vi "nodemcu_temp 00.vi"() -> ()   [LabVIEW 2018]
panel:
  out "웨이브폼 차트":dynamicdata(graph)
  out "Temp 2 (℃)":string
  out "온도2":dbl(graph)
  in  "문자열":string="http://192.168.137.202"
  out "Run":i32
  out "위치":path
  out "Data":string
  in  "불리언 2":bool=TRUE
  in  "Error In":errorcluster caption="에러 입력"
  out "Error Out":errorcluster caption="에러 출력"
  in  "정지 2":bool
  in  "Delay(s)":u32=4
  in  "188":bool=TRUE
  out "Temp 1 (℃)":string
  out "온도1":dbl(graph)
  in  "Clear":bool
  in  "정지":bool
  # "Temperture monitor"
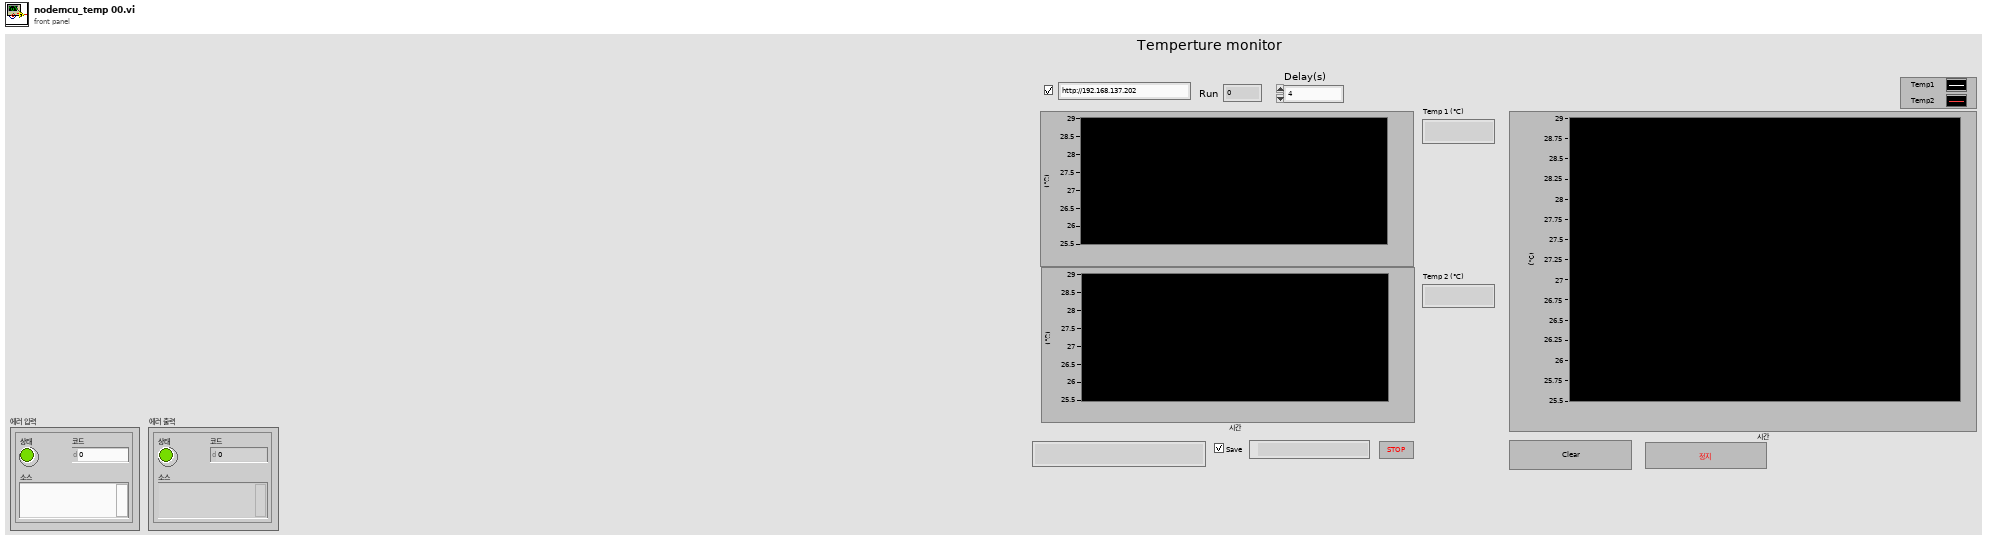
[diagram p1: front panel]
types:
  T1 = enum16{"Read", "Write", "ReadWrite", "BufferedRead", "BufferedReadWrite"}
  T2 = enum16{"open", "replace", "create", "open or create", "replace or create", "replace or create with confirmation"}
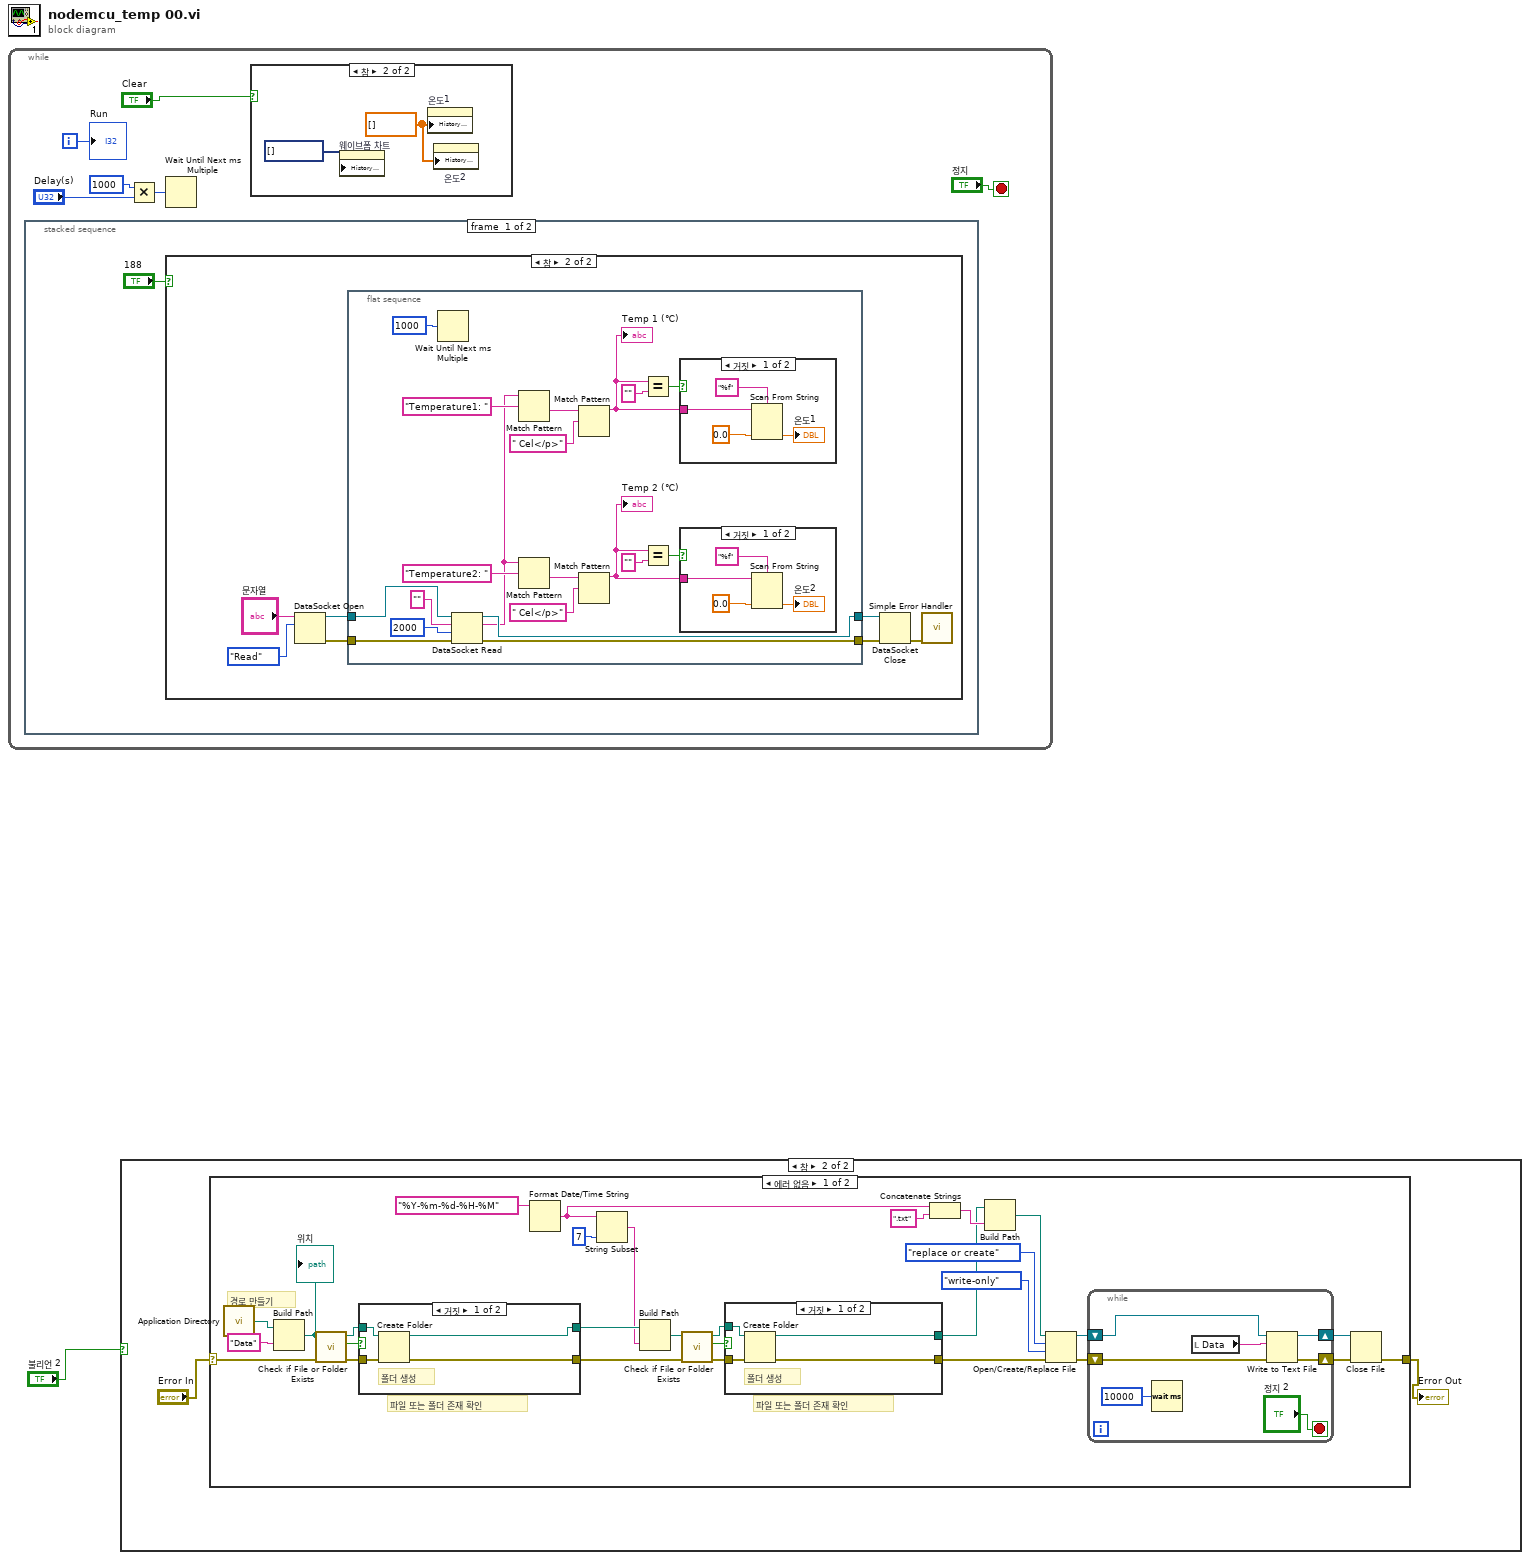
[diagram p0: block diagram]
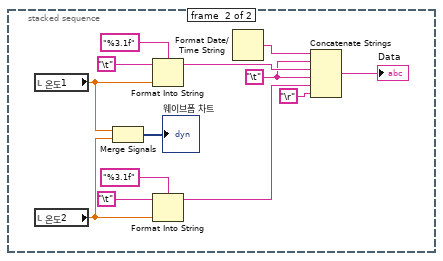
[diagram p10: hidden frame]
diagram:
  n1 = while {
    i -> [w5]
    stop <- "정지" stop-if-true
    n2 = stacked-sequence {
      frame #0 {
        n3 = case shown="참" "188" {
          frame False {
          }
          frame True {
            n4 = DataSocket Open(10:T1."Read" ("mode"), 11:"문자열") -> (0:w13:errorcluster, 3:w15:refnum<k13>)  [unwired: 2 in]
            n5 = flat-sequence {
              tunnel: w15 -> [w37]
              tunnel: [w36] -> w14
              tunnel: w13 -> [w35]
              tunnel: [w34] -> w12
              frame #0 {
                n6 = Wait Until Next ms Multiple(millisecond multiple=u32 1000 ("ms 배수")) -> ()  [unwired: 1 out]
                n7 = DataSocket Read(8:w35, 9:2000 ("ms 타임아웃(10000)"), 10:"", 11:w37) -> (0:w34:errorcluster, 2:w18:string, 3:w36:refnum<k13>)  [unwired: 1 in, 4 out]
                n8 = Match Pattern(string=w18, regular expression="Temperature1: " ("검색 문자열/문자 (-)")) -> (after substring=w33:string)  [unwired: 1 in, 3 out]
                n9 = Match Pattern(string=w18, regular expression="Temperature2: " ("검색 문자열/문자 (-)")) -> (after substring=w19:string)  [unwired: 1 in, 3 out]
                n10 = Match Pattern(string=w33, regular expression=" Cel</p>" ("정규식")) -> (before substring=w26:string)  [unwired: 1 in, 3 out]
                "Temp 1 (℃)" <- w26
                n11 = Match Pattern(string=w19, regular expression=" Cel</p>" ("정규식")) -> (before substring=w24:string)  [unwired: 1 in, 3 out]
                "Temp 2 (℃)" <- w24
                n12 = Equal?(x=w26, y="") -> (x = y?=w27:bool)
                n13 = Equal?(x=w24, y="") -> (x = y?=w23:bool)
                n14 = case shown="거짓" w27 {
                  tunnel: w26 -> [w42 _]
                  frame False {
                    n15 = Scan From String(format string="%f" ("포맷 문자열"), input string=w42, default 1=0.0 ("기본값 1")) -> (output 1=→"온도1":dbl)  [unwired: 2 in, 3 out]
                  }
                  frame True {
                  }
                }
                n16 = case shown="거짓" w23 {
                  tunnel: w24 -> [w38 _]
                  frame False {
                    n17 = Scan From String(format string="%f" ("포맷 문자열"), input string=w38, default 1=0.0 ("기본값 1")) -> (output 1=→"온도2":dbl)  [unwired: 2 in, 3 out]
                  }
                  frame True {
                  }
                }
              }
            }
            n18 = DataSocket Close(8:w12, 11:w14) -> (0:w16:errorcluster)  [unwired: 1 in, 1 out]
            n19 = call <vilib>:"Simple Error Handler.vi"("error in (no error)"=w16) -> ()  [unwired: 4 in, 5 out]
          }
        }
      }
      frame #1 {
        w49 = "\t"
        n20 = local read "온도1"() -> (w48:dbl)
        n21 = local read "온도2"() -> (w47:dbl)
        n22 = Merge Signals(w48, w47) -> (→"웨이브폼 차트":dynamicdata)
        n23 = Format Into String(format string="%3.1f" ("포맷 문자열"), initial string="\t", w48) -> (resulting string=w57:string)  [unwired: 1 in, 1 out]
        n24 = Format Into String(format string="%3.1f" ("포맷 문자열"), initial string="\t", w47) -> (resulting string=w50:string)  [unwired: 1 in, 1 out]
        n25 = Format Date/Time String() -> (date/time string=w55:string)  [unwired: 3 in]
        n26 = Concatenate Strings(w55, w49, w57, w49, w50, "\r") -> (→"Data":string)
      }
    }
    n27 = Multiply(x=u32 1000 ("ms 배수"), y="Delay(s)") -> (x*y=w4:u32)
    n28 = Wait Until Next ms Multiple(millisecond multiple=w4) -> ()  [unwired: 1 out]
    n29 = case shown="참" "Clear" {
      frame False {
      }
      frame True {
        w9 = dbl[] [] ("히스토리 데이터")
        n30 = property on="웨이브폼 차트" class="WFChart (엄격한)"("History Data"=dynamicdata[] [] ("히스토리 데이터")) -> ()  [unwired: 2 in, 2 out]
        n31 = property on="온도1" class="WFChart (엄격한)"("History Data"=w9) -> ()  [unwired: 2 in, 2 out]
        n32 = property on="온도2" class="WFChart (엄격한)"("History Data"=w9) -> ()  [unwired: 2 in, 2 out]
      }
    }
    "Run" <- w5
  }
  n33 = case shown="참" "불리언 2" {
    frame False {
    }
    frame True {
      n34 = case shown="에러 없음" "Error In" {
        selector: "Error In" -> [w89 w109]
        tunnel: [w73 w109] -> w59
        frame No Error {
          # "파일 또는 폴더 존재 확인"
          # "경로 만들기"
          # "파일 또는 폴더 존재 확인"
          n35 = call <vilib>:"Application Directory.vi"() -> ("Application Directory"=w88:path)
          n36 = Build Path(base path=w88, name or relative path="Data" ("이름 또는 상대 경로")) -> (appended path=w86:path)
          "위치" <- w86
          n37 = call <vilib>:"Check if File or Folder Exists.vi"("error in (no error)"=w89, "path"=w86) -> ("error out"=w85:errorcluster, "file or folder exists?"=w84:bool, "dup path"=w83:path)  [unwired: 7 in]
          n38 = case shown="거짓" w84 {
            tunnel: w85 -> [w105 w107]
            tunnel: w83 -> [w106 w108]
            tunnel: [w103 w108] -> w71
            tunnel: [w104 w107] -> w65
            frame False {
              # "폴더 생성"
              n39 = Create Folder(path (use dialog)=w106, error in=w105) -> (created path=w103:path, error out=w104:errorcluster)  [unwired: 1 in, 1 out]
            }
            frame True {
            }
          }
          n40 = Format Date/Time String(time format string (%c)="%Y-%m-%d-%H-%M" ("시간 포맷 문자열 (%c)")) -> (date/time string=w61:string)  [unwired: 2 in]
          n41 = String Subset(string=w61, length (rest)=7 ("길이(나머지)")) -> (substring=w70:string)  [unwired: 1 in]
          n42 = Build Path(base path=w71, name or relative path=w70) -> (appended path=w66:path)
          n43 = call <vilib>:"Check if File or Folder Exists.vi"("error in (no error)"=w65, "path"=w66) -> ("error out"=w67:errorcluster, "file or folder exists?"=w68:bool, "dup path"=w69:path)  [unwired: 7 in]
          n44 = case shown="거짓" w68 {
            tunnel: w67 -> [w99 w101]
            tunnel: w69 -> [w100 w102]
            tunnel: [w97 w102] -> w63
            tunnel: [w98 w101] -> w64
            frame False {
              # "폴더 생성"
              n45 = Create Folder(path (use dialog)=w100, error in=w99) -> (created path=w97:path, error out=w98:errorcluster)  [unwired: 1 in, 1 out]
            }
            frame True {
            }
          }
          n46 = Concatenate Strings(w61, ".txt" ("문자열")) -> (w75:string)
          n47 = Build Path(base path=w63, name or relative path=w75) -> (appended path=w74:path)
          n48 = Open/Create/Replace File(file path (use dialog)=w74, error in=w64, operation (0:open)=T2."replace or create" ("동작(0:open)"), access (0:read/write)=enum16{"read/write", "read-only", "write-only"}."write-only" ("접근(0:읽기/쓰기)")) -> (refnum out=w80:refnum<file>, error out=w79:errorcluster)  [unwired: 2 in, 1 out]
          n49 = while {
            shift-right: [w94] -> w78
            shift-left: w80 -> [w96]
            shift-right: [w93] -> w77
            shift-left: w79 -> [w95]
            stop <- "정지 2" stop-if-true
            n50 = Wait (ms)(milliseconds to wait=u32 10000 ("대기 시간 (ms)")) -> ()  [unwired: 1 out]
            n51 = local read "Data"() -> (w91:string)
            n52 = Write to Text File(file (use dialog)=w96, text=w91, error in=w95) -> (refnum out=w94:refnum<file>, error out=w93:errorcluster)  [unwired: 1 in, 1 out]
          }
          n53 = Close File(refnum=w78, error in=w77) -> (error out=w73:errorcluster)  [unwired: 1 out]
        }
        frame Error {
        }
      }
      "Error Out" <- w59
    }
  }
